vi "Exchange_dot-ID_All_Conn_Dots-1.vi"(4 "Minimal ID":u16, 5 "N (all dots in frame)":i32, 6 "ID-dot col IN":u16[](array[numeric]), 7 "multiplier(x4)":i32, 8 "Amount":i32, 9 "Indexes Conn Dot":i32[](array[numeric]), 10 "(X,Y...)-col":dbl[](array[numeric]), 11 "Statuses (col)":i16[](array[numeric])) -> (1 "Minimal ID OUT":u16, 2 "ID-dot col OUT":u16[](array[numeric]))   [LabVIEW 2013]
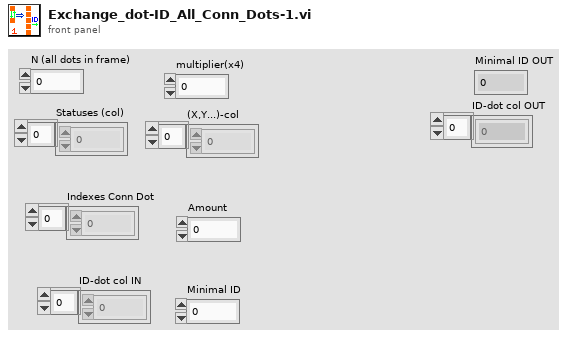
[diagram p1: front panel]
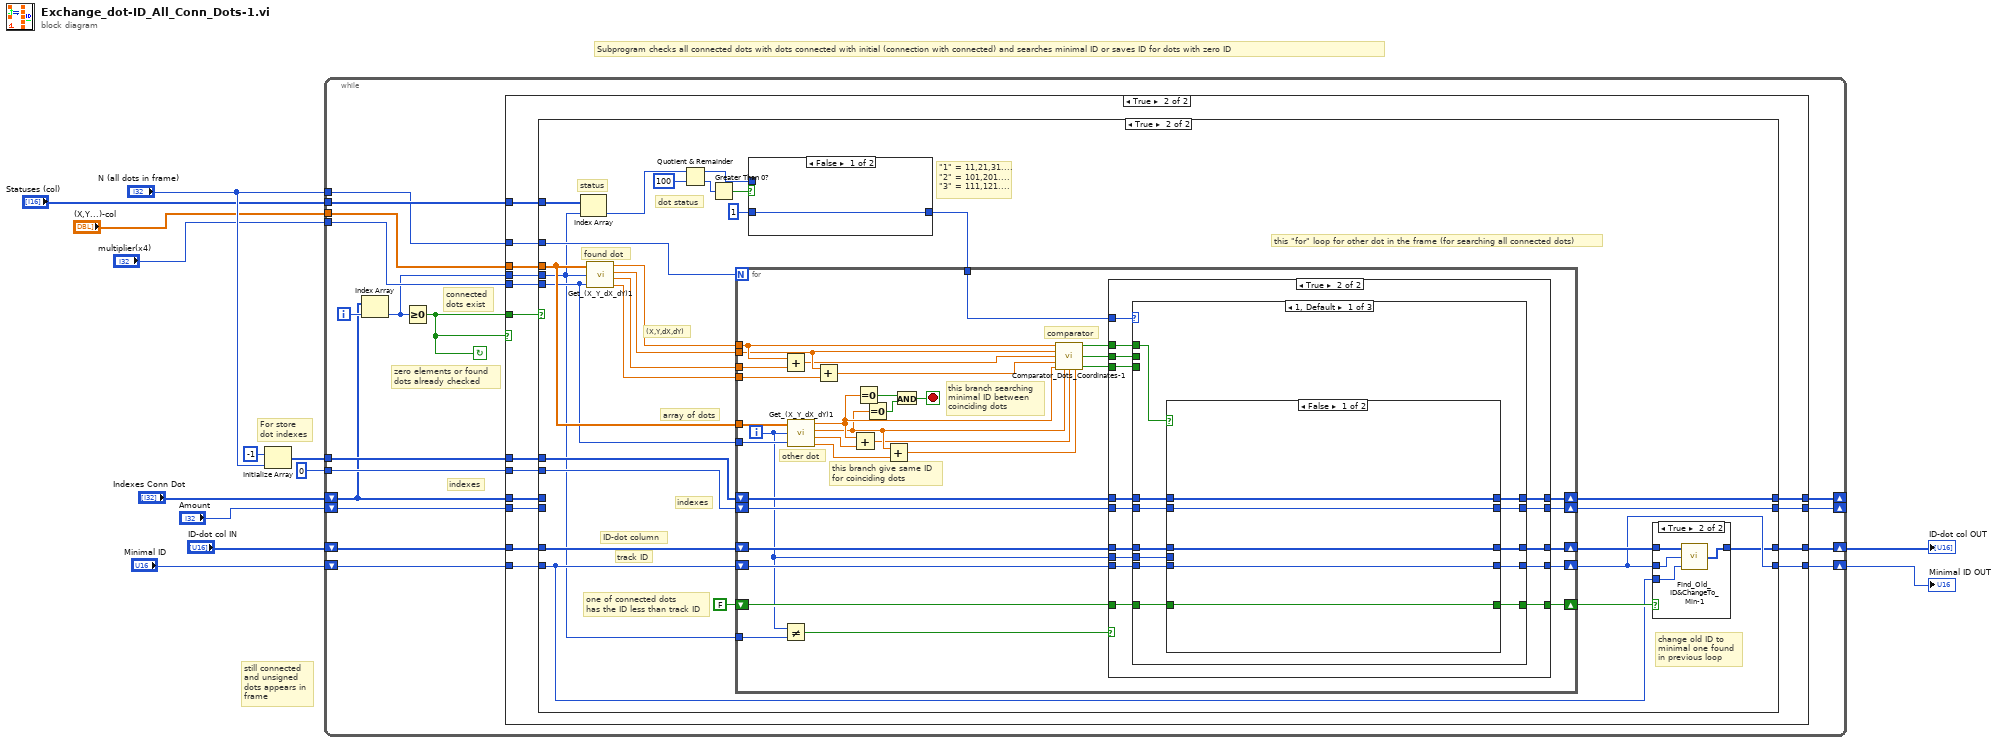
[diagram p0: block diagram]
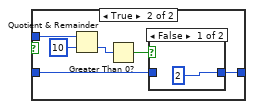
[diagram p4: hidden frame]
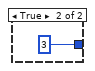
[diagram p5: hidden frame]
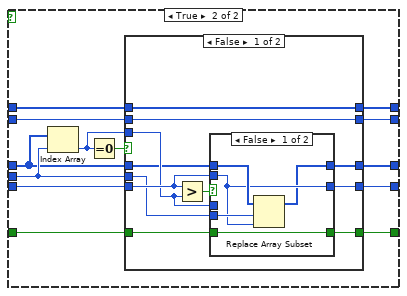
[diagram p8: hidden frame]
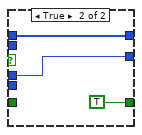
[diagram p9: hidden frame]
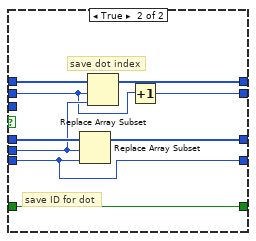
[diagram p10: hidden frame]
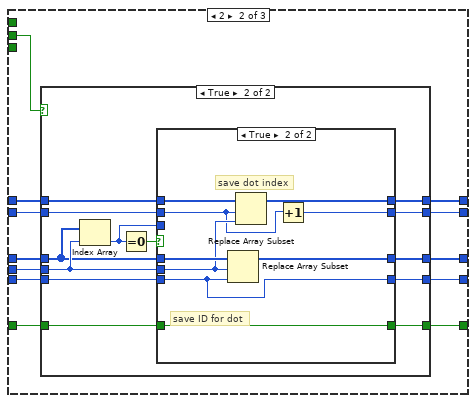
[diagram p11: hidden frame]
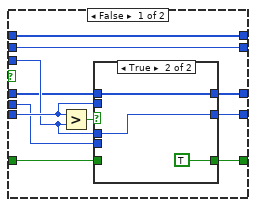
[diagram p13: hidden frame]
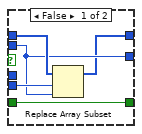
[diagram p14: hidden frame]
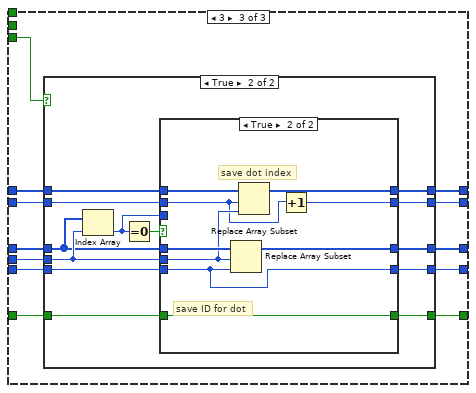
[diagram p15: hidden frame]
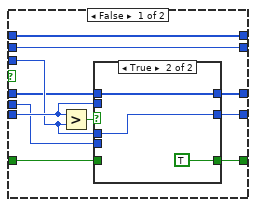
[diagram p17: hidden frame]
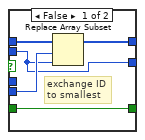
[diagram p18: hidden frame]
diagram:
  # "still connected \nand unsigned \ndots appears in\nframe"
  # "For store \ndot indexes"
  # "Subprogram checks all connected dots with dots connected with initial (connection with connected) and searches minimal ID or saves ID for dots with zero ID"
  n1 = Initialize Array(-1 ("element"), "N (all dots in frame)") -> (w2:i32[])
  n2 = while {
    shift-right: [w22] -> w4
    shift-left: "ID-dot col IN" -> [w30]
    shift-right: [w23] -> _
    shift-left: "Amount" -> [w19]
    shift-right: [w24] -> _
    shift-left: "Indexes Conn Dot" -> [w17]
    tunnel: "(X,Y...)-col" -> [w29]
    tunnel: "multiplier(x4)" -> [w28]
    tunnel: "Statuses (col)" -> [w27]
    tunnel: "N (all dots in frame)" -> [w26]
    tunnel: w2 -> [w21]
    tunnel: 0 -> [w20]
    shift-right: [w15] -> w5
    shift-left: "Minimal ID" -> [w25]
    i -> [w18]
    stop <- w14 continue-if-true
    # "indexes"
    # "connected\ndots exist"
    # "zero elements or found \ndots already checked"
    n3 = Index Array(array=w17, index=w18) -> (element=w16:i32)
    n4 = Greater Or Equal To 0?(x=w16) -> (x >= 0?=w14:bool)
    n5 = case shown="True" w14 {
      tunnel: w30 -> [w34 w50]
      tunnel: w17 -> [_ w39]
      tunnel: w29 -> [_ w49]
      tunnel: w28 -> [_ w48]
      tunnel: w27 -> [_ w46]
      tunnel: w26 -> [_ w47]
      tunnel: w25 -> [w31 w45]
      tunnel: [w33 w44] -> w24
      tunnel: [w32 w43] -> w23
      tunnel: [w34 w42] -> w22
      tunnel: w21 -> [w33 w41]
      tunnel: w20 -> [w32 w40]
      tunnel: w19 -> [_ w38]
      tunnel: w16 -> [_ w37]
      tunnel: w14 -> [_ w36]
      tunnel: [w31 w35] -> w15
      frame False {
      }
      frame True {
        n6 = case shown="True" w36 {
          tunnel: w50 -> [w54 w73]
          tunnel: w49 -> [_ w70]
          tunnel: w48 -> [_ w69]
          tunnel: w37 -> [_ w55]
          tunnel: w47 -> [_ w80]
          tunnel: w46 -> [_ w81]
          tunnel: w45 -> [w51 w65]
          tunnel: [w53 w72] -> w44
          tunnel: [w52 w71] -> w43
          tunnel: [w54 w63] -> w42
          tunnel: w41 -> [_ w75]
          tunnel: w40 -> [_ w74]
          tunnel: w39 -> [w53 _]
          tunnel: w38 -> [w52 _]
          tunnel: [w51 w64] -> w35
          frame False {
          }
          frame True {
            # "\"1\" = 11,21,31....\n\"2\" = 101,201....\n\"3\" = 111,121...."
            # "dot status"
            # "change old ID to\nminimal one found\nin previous loop"
            # "track ID"
            # "indexes"
            # "ID-dot column"
            # "this \"for\" loop for other dot in the frame (for searching all connected dots)"
            # "one of connected dots\nhas the ID less than track ID"
            # "status"
            # "found dot"
            # "array of dots"
            # "(X,Y,dX,dY)"
            n7 = Index Array(array=w81, index=w55) -> (element=w57:i16)
            n8 = call "Get_(X_Y_dX_dY)1.vi"("(X,Y,dX,dY)"=w70, "index"=w55, "multiplier"=w69) -> ("X"=w79:dbl, "Y"=w78:dbl, "dX"=w77:dbl, "dY"=w76:dbl)
            n9 = Quotient & Remainder(x=w57, y=i16 100) -> (x-y*floor(x/y)=w58:i16, floor(x/y)=w61:i16)
            n10 = Greater Than 0?(x=w61) -> (x > 0?=w60:bool)
            n11 = case shown="False" w60 {
              tunnel: 1 -> [w82 w84]
              tunnel: w58 -> [_ w88]
              tunnel: [w82 w83] -> w56
              frame False {
              }
              frame True {
                n12 = Quotient & Remainder(x=w88, y=i16 10) -> (floor(x/y)=w86:i16)  [unwired: 1 out]
                n13 = Greater Than 0?(x=w86) -> (x > 0?=w85:bool)
                n14 = case shown="False" w85 {
                  tunnel: w84 -> [_ _]
                  tunnel: [2 3] -> w83
                  frame False {
                  }
                  frame True {
                  }
                }
              }
            }
            n15 = for {
              N: w80 -> [_]
              tunnel: w70 -> [w129]
              tunnel: w69 -> [w123]
              tunnel: w79 -> [w113]
              tunnel: w78 -> [w112]
              tunnel: w77 -> [w122]
              tunnel: w76 -> [w121]
              shift-right: [w118] -> w66
              shift-left: w73 -> [w120]
              shift-right: [w115] -> w71
              shift-left: w74 -> [w116]
              shift-right: [w114] -> w72
              shift-left: w75 -> [w117]
              shift-right: [w102] -> w64
              shift-left: w65 -> [w119]
              shift-right: [w100] -> w67
              shift-left: FALSE -> [w101]
              tunnel: w56 -> [w99]
              tunnel: w55 -> [w97]
              i -> [w98]
              stop <- w126 stop-if-true
              # "this branch searching\nminimal ID between\ncoinciding dots"
              # "comparator"
              # "this branch give same ID \nfor coinciding dots"
              # "other dot"
              n16 = Add(x=w113, y=w122) -> (x+y=w111:dbl)
              n17 = Not Equal?(x=w98, y=w97) -> (x != y?=w96:bool)
              n18 = call "Get_(X_Y_dX_dY)1.vi"("(X,Y,dX,dY)"=w129, "index"=w98, "multiplier"=w123) -> ("X"=w109:dbl, "Y"=w108:dbl, "dX"=w125:dbl, "dY"=w124:dbl)
              n19 = Add(x=w112, y=w121) -> (x+y=w110:dbl)
              n20 = Add(x=w109, y=w125) -> (x+y=w107:dbl)
              n21 = Equal To 0?(x=w109) -> (x = 0?=w128:bool)
              n22 = Equal To 0?(x=w108) -> (x = 0?=w127:bool)
              n23 = Add(x=w108, y=w124) -> (x+y=w106:dbl)
              n24 = And(x=w128, y=w127) -> (x .and. y?=w126:bool)
              n25 = call "Comparator_Dots_Coordinates-1.vi"("X1"=w113, "Y1"=w112, "(X+dX)1"=w111, "(Y+dY)1"=w110, "X2"=w109, "Y2"=w108, "(X+dX)2"=w107, "(Y+dY)2"=w106) -> ("X1=X2,Y1=Y2 (1)"=w105:bool, "X1(2)=X2(2),Y1(2)=Y2(2) (2)"=w104:bool, "(1) OR (2) = (3)"=w103:bool)  [unwired: 5 in]
              n26 = case shown="True" w96 {
                tunnel: w120 -> [w132 w149]
                tunnel: w98 -> [_ w148]
                tunnel: w119 -> [w131 w147]
                tunnel: [w132 w146] -> w118
                tunnel: w117 -> [w134 w145]
                tunnel: w116 -> [w133 w144]
                tunnel: [w133 w143] -> w115
                tunnel: [w134 w142] -> w114
                tunnel: w105 -> [_ w141]
                tunnel: w104 -> [_ w140]
                tunnel: w103 -> [_ w139]
                tunnel: [w131 w138] -> w102
                tunnel: w101 -> [w130 w137]
                tunnel: [w130 w136] -> w100
                tunnel: w99 -> [_ w135]
                frame False {
                }
                frame True {
                  n27 = case shown="1, Default" w135 {
                    tunnel: w149 -> [w159 w216 w274]
                    tunnel: w148 -> [w158 w215 w273]
                    tunnel: w147 -> [w157 w214 w272]
                    tunnel: [w154 w210 w268] -> w146
                    tunnel: w145 -> [w161 w219 w277]
                    tunnel: w144 -> [w160 w218 w276]
                    tunnel: [w155 w211 w269] -> w143
                    tunnel: [w156 w212 w270] -> w142
                    tunnel: w141 -> [w153 _ _]
                    tunnel: w140 -> [_ w217 _]
                    tunnel: w139 -> [_ _ w275]
                    tunnel: [w152 w209 w267] -> w138
                    tunnel: w137 -> [w151 w213 w271]
                    tunnel: [w150 w208 w266] -> w136
                    frame 1, Default {
                      n28 = case shown="False" w153 {
                        tunnel: w159 -> [w166 w172]
                        tunnel: w158 -> [_ w173]
                        tunnel: w157 -> [w163 w179]
                        tunnel: [w166 w178] -> w154
                        tunnel: w161 -> [w165 w177]
                        tunnel: w160 -> [w164 w176]
                        tunnel: [w164 w175] -> w155
                        tunnel: [w165 w174] -> w156
                        tunnel: [w163 w169] -> w152
                        tunnel: w151 -> [w162 w168]
                        tunnel: [w162 w167] -> w150
                        frame False {
                        }
                        frame True {
                          n29 = Index Array(array=w172, index=w173) -> (element=w170:u16)
                          n30 = Equal To 0?(x=w170) -> (x = 0?=w171:bool)
                          n31 = case shown="False" w171 {
                            tunnel: w172 -> [w182 w207]
                            tunnel: w179 -> [w189 w200]
                            tunnel: [w180 w206] -> w178
                            tunnel: w177 -> [w186 w205]
                            tunnel: w173 -> [w181 w204]
                            tunnel: w176 -> [w185 w203]
                            tunnel: [w185 w202] -> w175
                            tunnel: [w186 w201] -> w174
                            tunnel: w170 -> [w187 _]
                            tunnel: [w188 w200] -> w169
                            tunnel: w168 -> [w184 w199]
                            tunnel: [w183 w199] -> w167
                            frame False {
                              n32 = Greater?(x=w189, y=w187) -> (0:w190:bool)
                              n33 = case shown="False" w190 {
                                tunnel: w189 -> [w192 _]
                                tunnel: [w192 w198] -> w188
                                tunnel: w187 -> [_ w198]
                                tunnel: w184 -> [w195 _]
                                tunnel: [w195 TRUE] -> w183
                                tunnel: w182 -> [w194 w196]
                                tunnel: w181 -> [w193 _]
                                tunnel: [w191 w196] -> w180
                                frame False {
                                n34 = Replace Array Subset(array=w194, new element=w192, index=w193) -> (w191:u16[])
                                }
                                frame True {
                                }
                              }
                            }
                            frame True {
                              # "save ID for dot"
                              # "save dot index"
                              n35 = Replace Array Subset(array=w207, new element=w200, index=w204) -> (w206:u16[])
                              n36 = Replace Array Subset(array=w205, new element=w204, index=w203) -> (w201:i32[])
                              n37 = Increment(x=w203) -> (x+1=w202:i32)
                            }
                          }
                        }
                      }
                    }
                    frame 2 {
                      n38 = case shown="True" w217 {
                        tunnel: w216 -> [w224 w230]
                        tunnel: w215 -> [_ w231]
                        tunnel: w214 -> [w221 w237]
                        tunnel: [w224 w236] -> w210
                        tunnel: w219 -> [w223 w235]
                        tunnel: w218 -> [w222 w234]
                        tunnel: [w222 w233] -> w211
                        tunnel: [w223 w232] -> w212
                        tunnel: [w221 w227] -> w209
                        tunnel: w213 -> [w220 w226]
                        tunnel: [w220 w225] -> w208
                        frame False {
                        }
                        frame True {
                          n39 = Index Array(array=w230, index=w231) -> (element=w228:u16)
                          n40 = Equal To 0?(x=w228) -> (x = 0?=w229:bool)
                          n41 = case shown="True" w229 {
                            tunnel: w230 -> [w240 w265]
                            tunnel: w237 -> [w247 w258]
                            tunnel: [w238 w264] -> w236
                            tunnel: w235 -> [w244 w263]
                            tunnel: w231 -> [w239 w262]
                            tunnel: w234 -> [w243 w261]
                            tunnel: [w243 w260] -> w233
                            tunnel: [w244 w259] -> w232
                            tunnel: w228 -> [w245 _]
                            tunnel: [w246 w258] -> w227
                            tunnel: w226 -> [w242 w257]
                            tunnel: [w241 w257] -> w225
                            frame False {
                              n42 = Greater?(x=w247, y=w245) -> (0:w248:bool)
                              n43 = case shown="True" w248 {
                                tunnel: w247 -> [w250 _]
                                tunnel: [w250 w256] -> w246
                                tunnel: w245 -> [_ w256]
                                tunnel: w242 -> [w253 _]
                                tunnel: [w253 TRUE] -> w241
                                tunnel: w240 -> [w252 w254]
                                tunnel: w239 -> [w251 _]
                                tunnel: [w249 w254] -> w238
                                frame False {
                                n44 = Replace Array Subset(array=w252, new element=w250, index=w251) -> (w249:u16[])
                                }
                                frame True {
                                }
                              }
                            }
                            frame True {
                              # "save ID for dot"
                              # "save dot index"
                              n45 = Replace Array Subset(array=w265, new element=w258, index=w262) -> (w264:u16[])
                              n46 = Replace Array Subset(array=w263, new element=w262, index=w261) -> (w259:i32[])
                              n47 = Increment(x=w261) -> (x+1=w260:i32)
                            }
                          }
                        }
                      }
                    }
                    frame 3 {
                      n48 = case shown="True" w275 {
                        tunnel: w274 -> [w282 w288]
                        tunnel: w273 -> [_ w289]
                        tunnel: w272 -> [w279 w295]
                        tunnel: [w282 w294] -> w268
                        tunnel: w277 -> [w281 w293]
                        tunnel: w276 -> [w280 w292]
                        tunnel: [w280 w291] -> w269
                        tunnel: [w281 w290] -> w270
                        tunnel: [w279 w285] -> w267
                        tunnel: w271 -> [w278 w284]
                        tunnel: [w278 w283] -> w266
                        frame False {
                        }
                        frame True {
                          n49 = Index Array(array=w288, index=w289) -> (element=w286:u16)
                          n50 = Equal To 0?(x=w286) -> (x = 0?=w287:bool)
                          n51 = case shown="True" w287 {
                            tunnel: w288 -> [w298 w323]
                            tunnel: w295 -> [w305 w316]
                            tunnel: [w296 w322] -> w294
                            tunnel: w293 -> [w302 w321]
                            tunnel: w289 -> [w297 w320]
                            tunnel: w292 -> [w301 w319]
                            tunnel: [w301 w318] -> w291
                            tunnel: [w302 w317] -> w290
                            tunnel: w286 -> [w303 _]
                            tunnel: [w304 w316] -> w285
                            tunnel: w284 -> [w300 w315]
                            tunnel: [w299 w315] -> w283
                            frame False {
                              n52 = Greater?(x=w305, y=w303) -> (0:w306:bool)
                              n53 = case shown="True" w306 {
                                tunnel: w305 -> [w308 _]
                                tunnel: [w308 w314] -> w304
                                tunnel: w303 -> [_ w314]
                                tunnel: w300 -> [w311 _]
                                tunnel: [w311 TRUE] -> w299
                                tunnel: w298 -> [w310 w312]
                                tunnel: w297 -> [w309 _]
                                tunnel: [w307 w312] -> w296
                                frame False {
                                # "exchange ID\nto smallest"
                                n54 = Replace Array Subset(array=w310, new element=w308, index=w309) -> (w307:u16[])
                                }
                                frame True {
                                }
                              }
                            }
                            frame True {
                              # "save ID for dot"
                              # "save dot index"
                              n55 = Replace Array Subset(array=w323, new element=w316, index=w320) -> (w322:u16[])
                              n56 = Replace Array Subset(array=w321, new element=w320, index=w319) -> (w317:i32[])
                              n57 = Increment(x=w319) -> (x+1=w318:i32)
                            }
                          }
                        }
                      }
                    }
                  }
                }
              }
            }
            n58 = case shown="True" w67 {
              tunnel: w66 -> [w91 w95]
              tunnel: w64 -> [_ w94]
              tunnel: w65 -> [_ w93]
              tunnel: [w91 w92] -> w63
              frame False {
              }
              frame True {
                n59 = call "Find_Old_ID&ChangeTo_Min-1.vi"("track ID OLD"=w93, "track ID (min)"=w94, "ID-dot col IN"=w95) -> ("ID-dot col OUT"=w92:u16[])
              }
            }
          }
        }
      }
    }
  }
  "Minimal ID OUT" <- w5
  "ID-dot col OUT" <- w4
